vi "StartStopServer.vi"() -> ()   [LabVIEW 2014]
panel:
  in  "Web Server:Server Active":bool
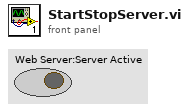
[diagram p1: front panel]
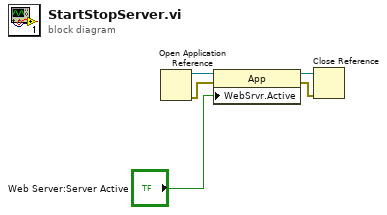
[diagram p0: block diagram]
diagram:
  n1 = Open Application Reference() -> (0:w2:errorcluster, 3:w5:refnum<vi>)  [unwired: 4 in]
  n2 = property class="App"(reference=w5, error in=w2, "WebSrvr.Active"="Web Server:Server Active") -> (reference out=w3:refnum<vi>, error out=w4:errorcluster)
  n3 = Close Reference(reference=w3, error in (no error)=w4) -> ()  [unwired: 1 out]
